vi "A33OutputOnOff.vi"(4 "Output mode (F:NORM,T:GATED)":bool, 5 "Enable Output (T: Enable)":bool=TRUE, 7 "Polarity (0: Normal)":u16(ring) items=["Normal", "Inverted"], 8 "error in (no error)":errorcluster, 9 "Impedance (50.0 Ohms)":dbl=50.0, 10 "Channel (1: Channel1)":u16(ring)=1 items=["Channel1"=1, "Channel2"=2], 11 "VISA resource name":refnum<visa-resource-name>) -> (0 "error out":errorcluster, 3 "VISA resource name out":refnum<visa-resource-name>)   [LabVIEW 2022 SP3]
doc: "Configures the output impedance and source impedance for the channel you specify."
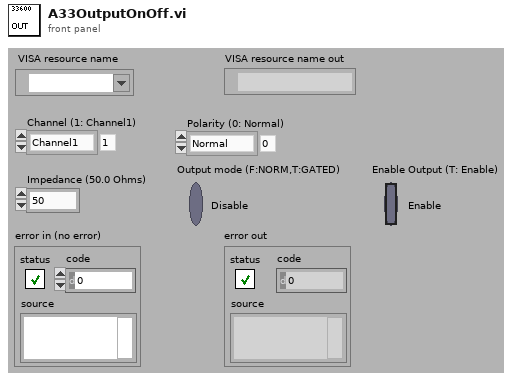
[diagram p1: front panel]
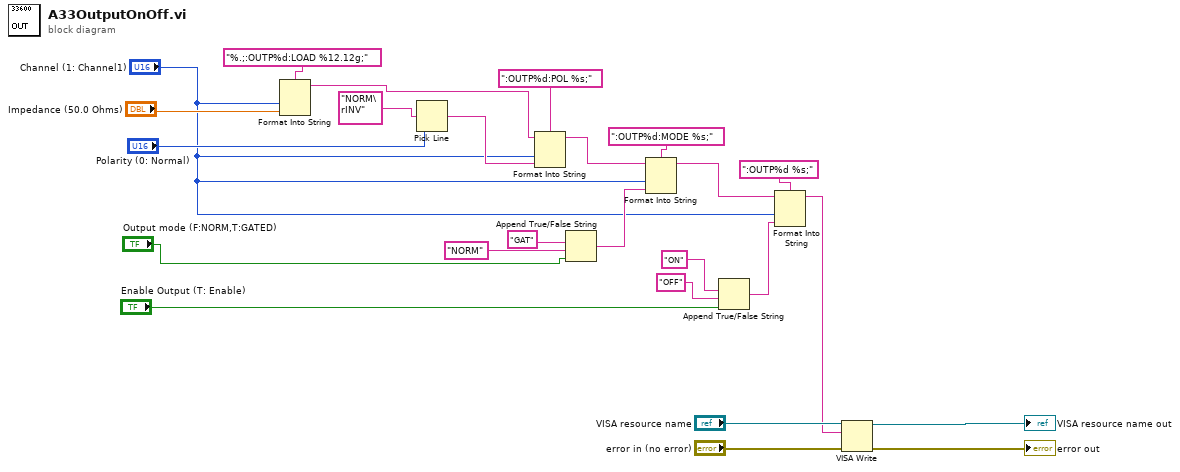
[diagram p0: block diagram]
diagram:
  n1 = Format Into String(format string="%.;:OUTP%d:LOAD %12.12g;", "Channel (1: Channel1)", "Impedance (50.0 Ohms)") -> (resulting string=w9:string)  [unwired: 2 in, 1 out]
  n2 = Pick Line(multi-line string="NORM\rINV", line index="Polarity (0: Normal)") -> (output string=w17:string)  [unwired: 1 in]
  n3 = Format Into String(format string=":OUTP%d:POL %s;", initial string=w9, "Channel (1: Channel1)", w17) -> (resulting string=w7:string)  [unwired: 1 in, 1 out]
  n4 = Append True/False String(1:"Output mode (F:NORM,T:GATED)", 2:"NORM" ("true string"), 3:"GAT" ("true string")) -> (0:w6:string)  [unwired: 1 in]
  n5 = Format Into String(format string=":OUTP%d:MODE %s;", initial string=w7, "Channel (1: Channel1)", w6) -> (resulting string=w4:string)  [unwired: 1 in, 1 out]
  n6 = Append True/False String(1:"Enable Output (T: Enable)", 2:"OFF" ("true string"), 3:"ON" ("true string")) -> (0:w2:string)  [unwired: 1 in]
  n7 = Format Into String(format string=":OUTP%d %s;", initial string=w4, "Channel (1: Channel1)", w2) -> (resulting string=w1:string)  [unwired: 1 in, 1 out]
  n8 = VISA Write(VISA resource name="VISA resource name", write buffer=w1, error in (no error)="error in (no error)") -> (VISA resource name out=→"VISA resource name out":refnum<visa-resource-name>, error out=→"error out":errorcluster)  [unwired: 1 out]
